vi "Get Selected Options.vi"(8 "error in":errorcluster, 10 "Menu":T1(array[cluster]), 11 "Changed Value":T2(array[cluster])) -> (0 "error out":errorcluster, 3 "Selected Option":string)   [LabVIEW 2019]
doc: "All Rights Reserved © 2017 SyncSols"
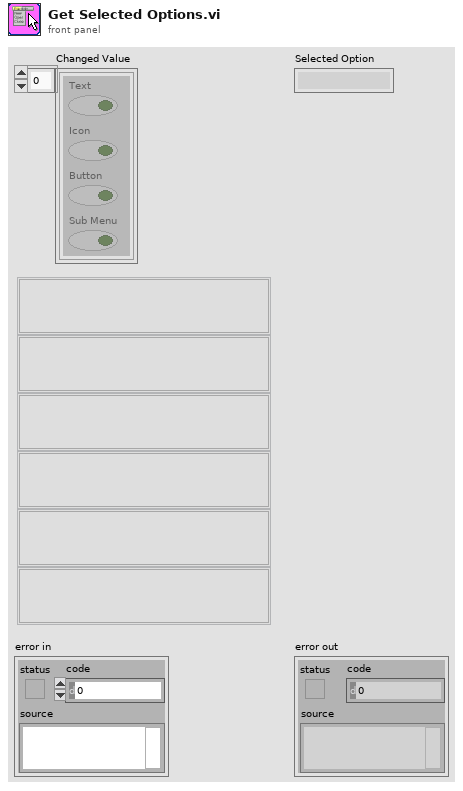
[diagram p1: front panel]
types:
  T1 = cluster{"Text ":string, "Icon":picture, "Button":bool, "Sub Menu":picture}[]
  T2 = cluster{"Text ":bool, "Icon":bool, "Button":bool, "Sub Menu":bool}[]
  T3 = cluster{"Text ":string, "Icon":picture, "Button":bool, "Sub Menu":picture}
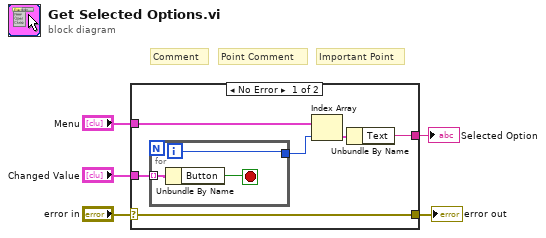
[diagram p0: block diagram]
diagram:
  # "Important Point"
  # "Point Comment"
  # "Comment"
  n1 = case shown="No Error" "error in" {
    selector: "error in" -> [w11 w15]
    tunnel: [w11 w15] -> w5
    tunnel: "Changed Value" -> [w10 _]
    tunnel: "Menu" -> [w8 _]
    tunnel: [w6 _] -> w1
    frame No Error {
      n2 = for {
        tunnel: w10 -> [w14] mode=indexing
        tunnel: [w12] -> w9
        i -> [w12]
        stop <- w13 stop-if-true
        n3 = Unbundle By Name(w14) -> ("Button"=w13:bool)
      }
      n4 = Index Array(array=w8, index=w9) -> (element=w7:T3)
      n5 = Unbundle By Name(w7) -> ("Text"=w6:string)
    }
    frame Error {
    }
  }
  "error out" <- w5
  "Selected Option" <- w1
